vi "Get Reply.vi"(0 "Socket":u32 format="%x", 1 "TxTimeStamp Alt":u32, 2 "ProcessID":u32 format="%04x", 11 "Error In":errorcluster, 12 "Timeout (ms)":i32) -> (4 "Ping Reply Info":T1 {"Sequence" format="%04x"}, 6 "RxBytes":i32 caption="Bytes\nReceived\nBack", 8 "RxCount":i32 caption="Packets Received", 10 "Timed Out?":bool, 15 "Error Out":errorcluster)   [LabVIEW 2018]
uses:
  Ping Reply Info.ctl
  Instance           8 17Saved   Get Reply .vi
panel:
  in  "Dump\nPacket\nto Disk\nfor\nDebug":bool
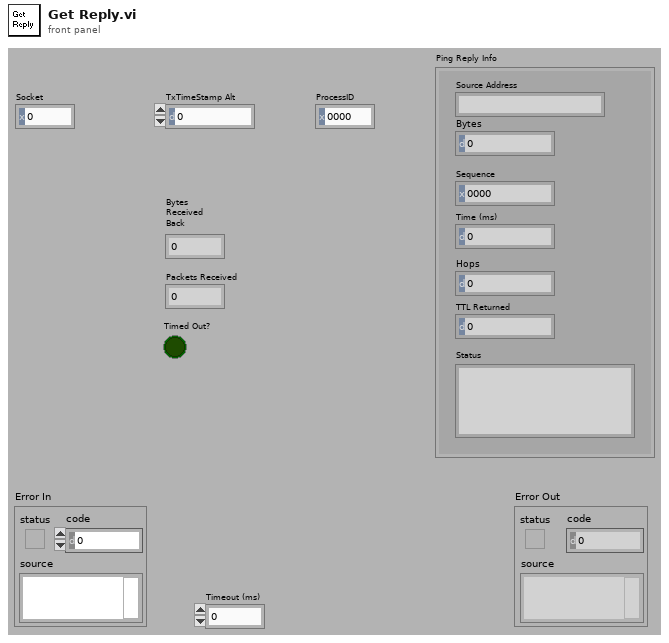
[diagram p1: front panel]
types:
  T1 = typedef "Ping Reply Info.ctl" = cluster{"Source Address":string, "Bytes":i32, "Sequence":u16, "Time (ms)":i32, "Hops":u8, "TTL Returned":u8, "Status":string}
  T2 = typedef "IP Packet Info.ctl" = cluster{"IP Version":u8, "IP Header Length (bytes)":u8, "Type of Service":u8, "ID":u16, "Flags":u8, "Total Length (Bytes)":u16, "Fragment Offset":u16, "TTL":u8, "Protocol ID":u8, "Header Checksum":u16, "Source Address":string, "Destination Address":string, "Options":u8[], "Data":u8[]}
  T3 = typedef "ICMP Packet Info.ctl" = cluster{"Type":u8, "Code":u8, "Checksum":u16, "ID":u16, "Sequence Number":u16, "TimeStamp":u32, "Data":u8[]}
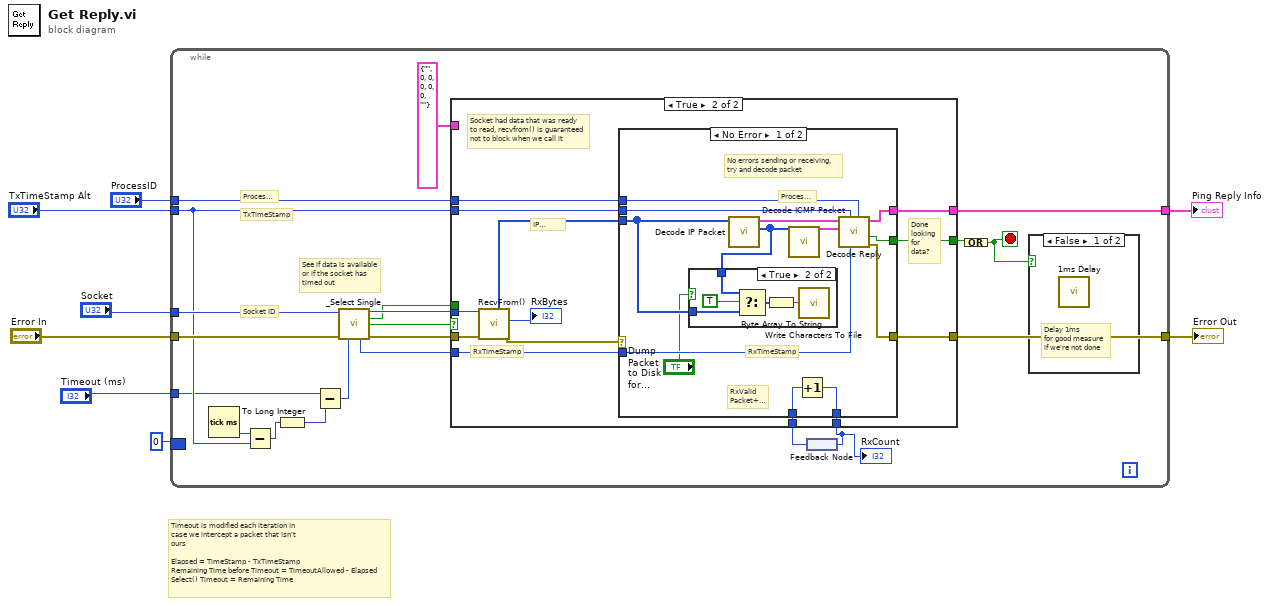
[diagram p0: block diagram]
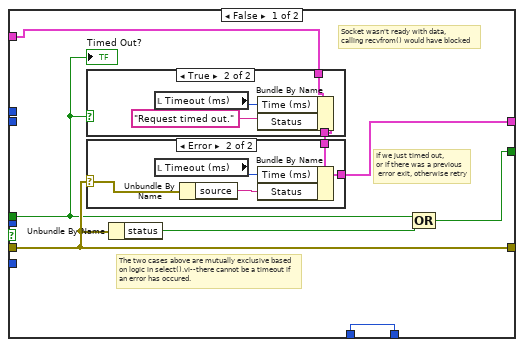
[diagram p2: hidden frame]
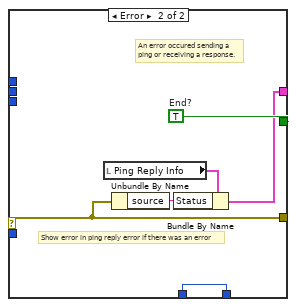
[diagram p6: hidden frame]
diagram:
  # "Timeout is modified each iteration in\ncase we intercept a packet that isn't\nours\n\nElapsed = TimeStamp - TxTimeStamp\nRemaining Time before Timeout = TimeoutAllowed - Elapsed\nSelect() Timeout = Remaining Time"
  n1 = while {
    tunnel: "Error In" -> [w24]
    tunnel: [w29] -> w6
    tunnel: "Socket" -> [w19]
    tunnel: [w28] -> w7
    tunnel: "ProcessID" -> [w27]
    tunnel: "TxTimeStamp Alt" -> [w14]
    tunnel: "Timeout (ms)" -> [w11]
    border: 0 ("RxCount") -> [_]
    stop <- w26 stop-if-true
    # "TxTimeStamp"
    # "Socket ID"
    # "ProcessID"
    # "See if data is available\nor if the socket has \ntimed out"
    n2 = Tick Count (ms)() -> (millisecond timer value=w13:u32)
    n3 = Subtract(x=w13, y=w14) -> (x-y=w21:u32)
    n4 = To Long Integer(number=w21) -> (32bit integer=w22:i32)
    n5 = Subtract(x=w11, y=w22) -> (x-y=w12:i32)
    n6 = call "_Select Single.vi"("Socket"=w19, "Error In"=w24, "Timeout (ms)"=w12) -> ("Socket Out"=w25:u32, "Timeout?"=w16:bool, "Socket Ready?"=w18:bool, "RxTimeStamp"=w15:u32, "Error Out"=w23:errorcluster)  [unwired: 8 in]
    n7 = feedback #1() -> (w10:i32)
    n8 = case shown="True" w18 {
      tunnel: [w35 w61] -> w29
      tunnel: [w32 w59] -> w28
      tunnel: w27 -> [_ w58]
      tunnel: [w37 w56] -> w20
      tunnel: w25 -> [_ w55]
      tunnel: w23 -> [w35 w54]
      tunnel: w16 -> [w31 _]
      tunnel: w14 -> [_ w53]
      tunnel: w15 -> [_ w52]
      tunnel: T1 {"Source Address"="", "Bytes"=0, "Sequence"=0, "Time (ms)"=0, "Hops"=0, "TTL Returned"=0, "Status"=""} ("Ping Reply Info") -> [w33 _]
      tunnel: w10 -> [w30 w51]
      tunnel: [w30 w50] -> w9
      frame False {
        # "The two cases above are mutually exclusive based\non logic in select().vi--there cannot be a timeout if\nan error has occured."
        # "If we just timed out, \nor if there was a previous\n error exit, otherwise retry"
        # "Socket wasn't ready with data,\ncalling recvfrom() would have blocked"
        n9 = case shown="True" w31 {
          tunnel: [w44 w48] -> w34
          tunnel: w33 -> [w44 w47]
          frame False {
          }
          frame True {
            n10 = local read "Timeout (ms)"() -> (w45:i32)
            n11 = Bundle By Name(cluster=w47, "Time (ms)"=w45, "Status"="Request timed out.") -> (w48:T1)
          }
        }
        n12 = case shown="Error" w35 {
          selector: w35 -> [_ w40]
          tunnel: w34 -> [w38 w42]
          tunnel: [w38 w41] -> w32
          frame No Error {
          }
          frame Error {
            n13 = local read "Timeout (ms)"() -> (w39:i32)
            n14 = Unbundle By Name(w40) -> ("source"=w43:string)
            n15 = Bundle By Name(cluster=w42, "Time (ms)"=w39, "Status"=w43) -> (w41:T1)
          }
        }
        n16 = Unbundle By Name(w35) -> ("status"=w36:bool)
        n17 = Compound Arithmetic op=OR(w31, w36) -> (w37:bool)
        "Timed Out?" <- w31
      }
      frame True {
        # "RxTimeStamp"
        # "Done\nlooking\nfor\ndata?"
        # "Socket had data that was ready\nto read, recvfrom() is guaranteed\nnot to block when we call it"
        # "IP Packet"
        n18 = call "RecvFrom().vi"("Error In"=w54, "Socket To Use"=w55) -> ("Error Out"=w60:errorcluster, "Bytes Read"=→"RxBytes":i32, "Received IP Packet"=w57:u8[])  [unwired: 4 in, 3 out]
        n19 = case shown="No Error" w60 {
          selector: w60 -> [_ w84]
          tunnel: w57 -> [w67 _]
          tunnel: [w62 w84] -> w61
          tunnel: [w72 w83] -> w59
          tunnel: [w63 w85] -> w56
          tunnel: w58 -> [w71 _]
          tunnel: w53 -> [w70 _]
          tunnel: w52 -> [w69 _]
          tunnel: w51 -> [w65 w80]
          tunnel: [w64 w80] -> w50
          frame No Error {
            # "RxValid\nPacket+=1"
            # "RxTimeStamp"
            # "ProcessID"
            # "No errors sending or receiving, \ntry and decode packet"
            n20 = call "Decode IP Packet.vi"("IP Packet"=w67) -> ("Data Out"=w68:u8[], "IP Packet"=w73:T2)  [unwired: 9 in]
            n21 = case shown="True" "Dump\nPacket\nto Disk\nfor\nDebug" {
              tunnel: w68 -> [_ w77]
              tunnel: w67 -> [_ w76]
              frame False {
              }
              frame True {
                n22 = Select(t=w77, s=TRUE, f=w76) -> (s? t:f=w78:u8[])
                n23 = Byte Array To String(unsigned byte array=w78) -> (string=w79:string)
                n24 = call <vilib>:"Write Characters To File.vi"("character string"=w79) -> ()  [unwired: 4 in, 1 out]
              }
            }
            n25 = call "Decode ICMP Packet.vi"("ICMP Packet"=w68) -> ("ICMP Packet Info"=w74:T3)  [unwired: 9 in, 1 out]
            n26 = Increment(x=w65) -> (x+1=w64:i32)
            n27 = call "Decode Reply.vi"("ProcessID"=w71, "RxTimeStamp"=w69, "TxTimeStamp Alt"=w70, "ICMP Packet Info"=w74, "IP Packet"=w73) -> ("Error Out"=w62:errorcluster, "Done?"=w63:bool, "Ping Reply Info"=w72:T1)  [unwired: 4 in]
          }
          frame Error {
            w85 = TRUE  # End?
            # "Show error in ping reply error if there was an error"
            # "An error occured sending a \nping or receiving a response."
            n28 = local read "Ping Reply Info"() -> (w82:T1)
            n29 = Unbundle By Name(w84) -> ("source"=w81:string)
            n30 = Bundle By Name(cluster=w82, "Status"=w81) -> (w83:T1)
          }
        }
      }
    }
    "RxCount" <- w9
    n31 = feedback-in #1(w9) -> ()
    n32 = Compound Arithmetic op=OR(w20) -> (w26:bool)
    n33 = case shown="False" w26 {
      frame False {
        # "Delay 1ms\nfor good measure\nif we're not done"
        n34 = call "1ms Delay"() -> ()  [unwired: 11 in, 1 out]
      }
      frame True {
      }
    }
  }
  "Error Out" <- w6
  "Ping Reply Info" <- w7
